vi "CRYView Pic WAIT GRAPH VI.vi"(10 "vi reference":refnum<vi>, 11 "sAction":string) -> (1 "sData_Out":string)   [LabVIEW 2013]
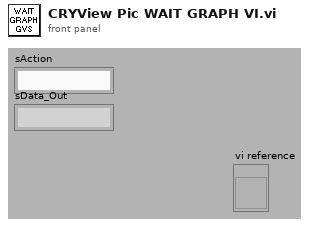
[diagram p1: front panel]
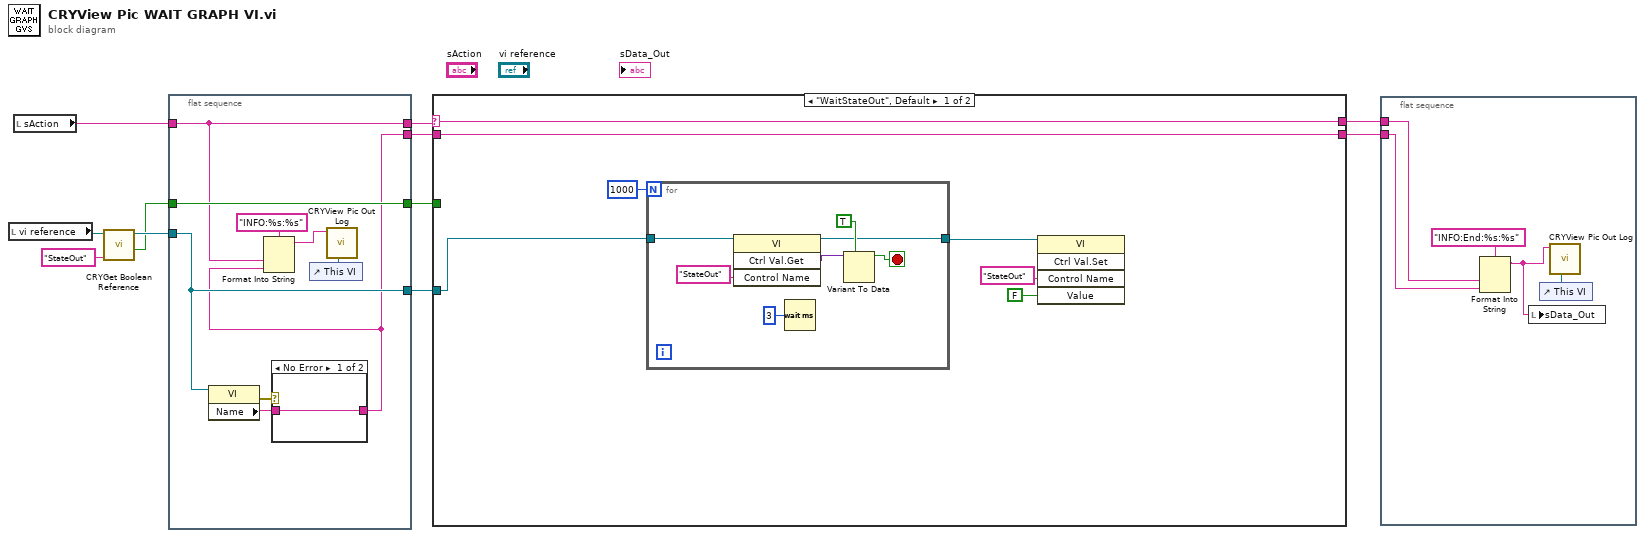
[diagram p0: block diagram]
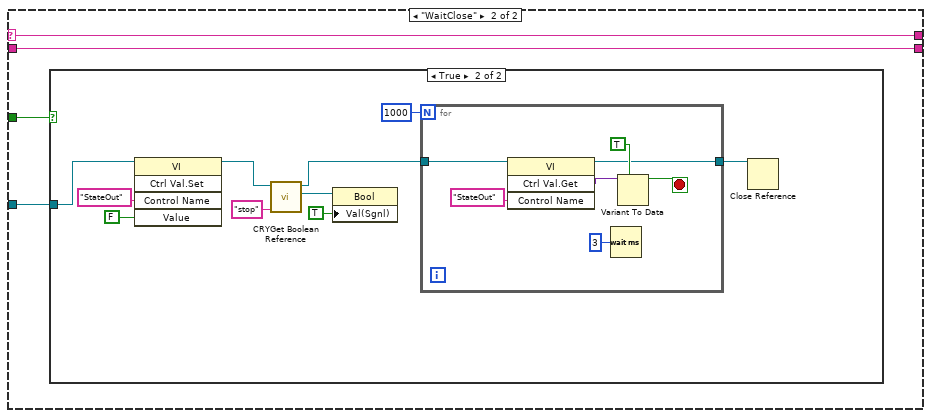
[diagram p2: hidden frame]
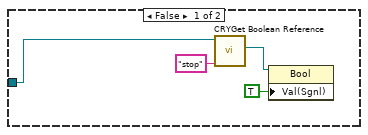
[diagram p3: hidden frame]
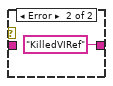
[diagram p4: hidden frame]
diagram:
  n1 = local read "vi reference"() -> (w6:refnum<vi>)
  n2 = local read "sAction"() -> (w5:string)
  n3 = call "CRYGet Boolean Reference.vi"("Label Name"="StateOut", "VI Refnum"=w6) -> ("Exist?"=w9:bool, "VI Refnum Out"=w10:refnum<vi>)  [unwired: 7 in, 1 out]
  n4 = flat-sequence {
    tunnel: [w16] -> w8
    tunnel: w10 -> [w16]
    tunnel: [w20] -> w7
    tunnel: w9 -> [w20]
    tunnel: w5 -> [w15]
    tunnel: [w15] -> w4
    tunnel: [w14] -> w2
    frame #0 {
      n5 = property class="VI"(reference=w16) -> (error out=w18:errorcluster, "Name"=w17:string)  [unwired: 1 in, 1 out]
      n6 = case shown="No Error" w18 {
        tunnel: w17 -> [w21 _]
        tunnel: [w21 "KilledVIRef" ("sAction")] -> w14
        frame No Error {
        }
        frame Error {
        }
      }
      n7 = Format Into String(format string="INFO:%s:%s" ("string"), w15, w14) -> (resulting string=w12:string)  [unwired: 2 in, 1 out]
      n8 = control-ref of="This VI"() -> (w13:refnum<vi>)
      n9 = call "CRYView Pic Out Log.vi"("vi reference"=w13, "sData"=w12) -> ()  [unwired: 10 in]
    }
  }
  n10 = case shown="\"WaitStateOut\", Default" w4 {
    selector: w4 -> [w29 w38]
    tunnel: w8 -> [w28 w40]
    tunnel: w7 -> [_ w39]
    tunnel: [w29 w38] -> w3
    tunnel: w2 -> [w27 w37]
    tunnel: [w27 w37] -> w1
    frame "WaitStateOut", Default {
      n11 = for {
        N: 1000 -> [_]
        tunnel: w28 -> [w35]
        tunnel: [w31] -> w24
        stop <- w30 stop-if-true
        n12 = invoke class="VI" method="Ctrl Val.Get"(reference=w35, "Control Name"="StateOut") -> (reference out=w31:refnum<vi>, "Get Control Value Variant"=w34:variant)  [unwired: 2 in, 2 out]
        n13 = Wait (ms)(milliseconds to wait=u32 3) -> ()  [unwired: 1 out]
        n14 = Variant To Data(type=TRUE, Variant=w34) -> (data=w30:bool)  [unwired: 1 in, 1 out]
      }
      n15 = invoke class="VI" method="Ctrl Val.Set"(reference=w24, "Control Name"="StateOut", "Value"=FALSE) -> ()  [unwired: 2 in, 5 out]
    }
    frame "WaitClose" {
      n16 = case shown="True" w39 {
        tunnel: w40 -> [w41 w47]
        frame False {
          n17 = call "CRYGet Boolean Reference.vi"("Label Name"="stop", "VI Refnum"=w41) -> ("Boolean Ref"=w44:refnum<vi>)  [unwired: 7 in, 2 out]
          n18 = property class="Bool"(reference=w44, "Val(Sgnl)"=TRUE) -> ()  [unwired: 1 in, 2 out]
        }
        frame True {
          n19 = invoke class="VI" method="Ctrl Val.Set"(reference=w47, "Control Name"="StateOut", "Value"=FALSE) -> (reference out=w49:refnum<vi>)  [unwired: 2 in, 4 out]
          n20 = call "CRYGet Boolean Reference.vi"("Label Name"="stop", "VI Refnum"=w49) -> ("Boolean Ref"=w52:refnum<vi>, "VI Refnum Out"=w48:refnum<vi>)  [unwired: 7 in, 1 out]
          n21 = property class="Bool"(reference=w52, "Val(Sgnl)"=TRUE) -> ()  [unwired: 1 in, 2 out]
          n22 = for {
            N: 1000 -> [_]
            tunnel: w48 -> [w60]
            tunnel: [w56] -> w46
            stop <- w55 stop-if-true
            n23 = invoke class="VI" method="Ctrl Val.Get"(reference=w60, "Control Name"="StateOut") -> (reference out=w56:refnum<vi>, "Get Control Value Variant"=w59:variant)  [unwired: 2 in, 2 out]
            n24 = Wait (ms)(milliseconds to wait=u32 3) -> ()  [unwired: 1 out]
            n25 = Variant To Data(type=TRUE, Variant=w59) -> (data=w55:bool)  [unwired: 1 in, 1 out]
          }
          n26 = Close Reference(reference=w46) -> ()  [unwired: 1 in, 1 out]
        }
      }
    }
  }
  n27 = flat-sequence {
    tunnel: w3 -> [w65]
    tunnel: w1 -> [w64]
    frame #0 {
      n28 = Format Into String(format string="INFO:End:%s:%s" ("string"), w65, w64) -> (resulting string=w62:string)  [unwired: 2 in, 1 out]
      n29 = local write "sData_Out"(w62) -> ()
      n30 = control-ref of="This VI"() -> (w63:refnum<vi>)
      n31 = call "CRYView Pic Out Log.vi"("vi reference"=w63, "sData"=w62) -> ()  [unwired: 10 in]
    }
  }
